vi "DeleteData.vi"(5 "FilesPath":path, 7 "Lista_Op_IN":refnum<vi>, 8 "error in":errorcluster, 9 "Value":i32, 10 "Item Names":string[](array[string]), 11 "Queues in":T1) -> (0 "error out":errorcluster, 3 "Queues out":T1)   [LabVIEW 2019]
uses:
  Queue/TypeDef/#TypeDef_App_Queues.ctl
  User Interface/TypeDef/#TypeDef_Enum_Buttons.ctl
  User Interface/TypeDef/#TypeDef_EventStructureConstant.ctl
  User Interface/TypeDef/#TypeDef_Enum_EventStructure.ctl
  Queue/TypeDef/#TypeDef_NetworkStream.ctl
  Communication/TypeDef/#TypeDef_FromMRtoPC.ctl
  Communication/TypeDef/#TypeDef_FromPCtoMR.ctl
  Communication/TypeDef/#TypeDef_Command.ctl
  Communication/TypeDef/#TypeDef_ErrorHandler_prop.ctl
  Communication/TypeDef/#TypeDef_PropGraph.ctl
  Communication/TypeDef/#TypeDef_PropertiesToSave.ctl
  <vilib>/addons/database/Connection.llb/Conn ObjectReference.ctl
  Test/TypeDef/#TypeDef_DataToTest.ctl
  Communication/TypeDef/#TypeDef_SetGet.ctl
  <vilib>/addons/database/NI_Database_API.lvlib
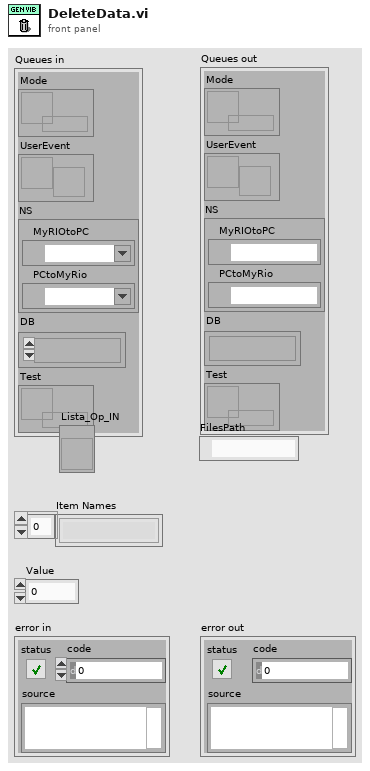
[diagram p1: front panel]
types:
  T1 = typedef "#TypeDef_App_Queues.ctl" = cluster{"Mode":refnum<queue>, "UserEvent":refnum<user-event>, "NS":T2, "DB":T3, "Test":refnum<queue>}
  T2 = typedef "#TypeDef_NetworkStream.ctl" = cluster{"MyRIOtoPC":refnum<k21>, "PCtoMyRio":refnum<k21>}
  T3 = typedef "NI_Database_API.lvlib/Conn ObjectReference.ctl" = refnum<k1>
  T4 = typedef "#TypeDef_SetGet.ctl" = enum16{"Set", "Get"}
  T5 = typedef "#TypeDef_DBMode.ctl" = u16
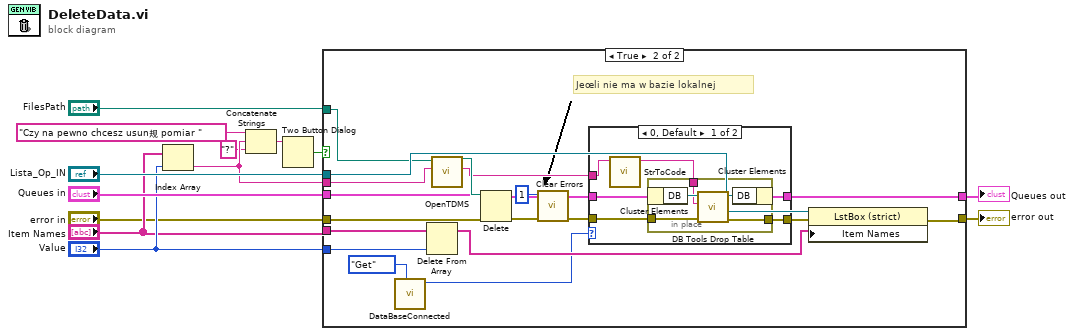
[diagram p0: block diagram]
diagram:
  n1 = Index Array(array="Item Names", index="Value") -> (element=w8:string)
  n2 = Concatenate Strings("Czy na pewno chcesz usun规 pomiar ", w8, "?" ("string")) -> (w4:string)
  n3 = Two Button Dialog(message=w4) -> (T button?=w5:bool)  [unwired: 2 in]
  n4 = case shown="True" w5 {
    tunnel: "error in" -> [w15 w32]
    tunnel: [w15 w28] -> w7
    tunnel: w8 -> [_ w31]
    tunnel: "Item Names" -> [_ w30]
    tunnel: "Value" -> [_ w29]
    tunnel: "Lista_Op_IN" -> [_ w26]
    tunnel: "Queues in" -> [w14 w25]
    tunnel: [w14 w24] -> w13
    tunnel: "FilesPath" -> [_ w23]
    frame False {
    }
    frame True {
      # "Jeœli nie ma w bazie lokalnej"
      n5 = call "DataBaseConnected.vi"("Get/Set"=#TypeDef_SetGet."Get") -> ("BD out"=w17:T5)  [unwired: 10 in]
      n6 = Delete From Array(array=w30, index=w29) -> (array with subset deleted=w27:string[])  [unwired: 1 in, 1 out]
      n7 = call "OpenTDMS.vi"("Name in"=w31, "FilesPath"=w23) -> ("Name out"=w16:string, "Path"=w33:path)  [unwired: 8 in]
      n8 = Delete(path (use dialog)=w33, error in=w32) -> (error out=w22:errorcluster)  [unwired: 3 in, 2 out]
      n9 = call <vilib>:"Clear Errors.vi"("error in (no error)"=w22, "specific error code to clear (0: all)"=1) -> ("error out"=w21:errorcluster)  [unwired: 4 in, 1 out]
      n10 = case shown="0, Default" w17 {
        tunnel: w25 -> [w39 w46]
        tunnel: [w38 w46] -> w24
        tunnel: w21 -> [w37 w45]
        tunnel: [w36 w45] -> w19
        tunnel: w16 -> [w35 _]
        frame 0, Default {
          n11 = call "StrToCode.vi"("Name in"=w35) -> ("Name out"=w34:string)  [unwired: 10 in]
          n12 = in-place {
            in-place-border: w37 -> [w42]
            in-place-border: [w41] -> w36
            in-place-border: w34 -> [w40]
            n13 = in-place-cluster #1(w39) -> ("DB"=w44:T3)
            n14 = call <vilib>:"DB Tools Drop Table.vi"("error in (no error)"=w42, "table"=w40, "connection reference"=w44) -> ("error out"=w41:errorcluster, "connection reference out"=w43:T3)  [unwired: 5 in]
            n15 = in-place-cluster #1("DB"=w43) -> (w38:T1)
          }
        }
        frame 1 {
        }
      }
      n16 = property class="LstBox (strict)"(reference=w26, error in=w19, "Item Names"=w27) -> (error out=w28:errorcluster)  [unwired: 1 out]
    }
  }
  "Queues out" <- w13
  "error out" <- w7
